vi "WPI_Power Get PDP EnergyPower.vi"(0 "Power Distribution Panel (0)":u8, 7 "Reset Energy?":bool, 11 "error in":errorcluster) -> (6 "Energy (J)":dbl, 8 "Power (W)":dbl, 15 "error out":errorcluster)   [LabVIEW 2017]
doc: "Return the Energy delivered to the robot as well as the recent power delivery."
uses:
  <vilib>/Rock Robotics/WPI/CAN/PDP/WPI_CAN_PDPGlobalOps.ctl
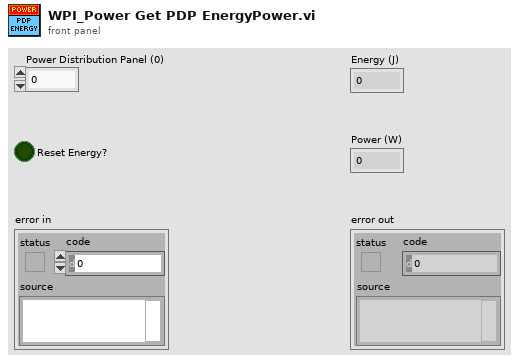
[diagram p1: front panel]
types:
  T1 = typedef "WPI_CAN_PDPGlobalOps.ctl" = enum16{"Write After Receive 0-5", "Write After Receive 6-11", "Write After Receive 12-15", "Write After Receive Energy", "Get All", "Get Commands", "Write Clear Sticky Faults Command", "Write Reset Energy Command", "Write Tare Currents Command", "Write Error", "Write After Receive Faults"}
  T2 = typedef "WPI_CAN_PDPGetAll.ctl" = cluster{"Channel Currents":dbl[], "Battery Voltage":dbl, "Temperature (degrees C)":dbl, "Internal Battery R (Ohms)":dbl, "Energy (J)":dbl, "Power (W)":dbl, "Total Current (A)":dbl, "CAN Error":errorcluster, "Current Faults":bool[], "Battery Voltage Fault":bool, "Temperature Fault":bool, "Hardware Fault":bool}
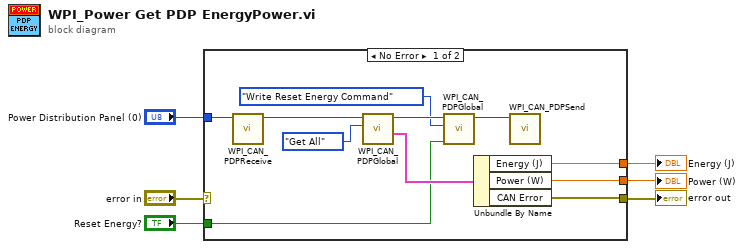
[diagram p0: block diagram]
diagram:
  n1 = case shown="No Error" "error in" {
    selector: "error in" -> [_ w18]
    tunnel: [w8 w18] -> w5
    tunnel: "Power Distribution Panel (0)" -> [w16 _]
    tunnel: [w7 _] -> w2
    tunnel: [w14 _] -> w3
    tunnel: "Reset Energy?" -> [w10 _]
    frame No Error {
      n2 = call <vilib>:"WPI_CAN_PDPReceive.vi"("Power Distribution Panel (0)"=w16) -> ("Power Distribution Panel Out"=w13:u8)  [unwired: 10 in]
      n3 = call <vilib>:"WPI_CAN_PDPGlobal.vi"("Operation"=WPI_CAN_PDPGlobalOps."Get All", "Power Distribution Panel (0)"=w13) -> ("Get All"=w17:T2, "Power Distribution Panel Out"=w12:u8)  [unwired: 7 in, 1 out]
      n4 = call <vilib>:"WPI_CAN_PDPGlobal.vi"("Command"=w10, "Operation"=WPI_CAN_PDPGlobalOps."Write Reset Energy Command", "Power Distribution Panel (0)"=w12) -> ("Power Distribution Panel Out"=w9:u8)  [unwired: 6 in, 2 out]
      n5 = Unbundle By Name(w17) -> ("Energy (J)"=w7:dbl, "Power (W)"=w14:dbl, "CAN Error"=w8:errorcluster)
      n6 = call <vilib>:"WPI_CAN_PDPSend.vi"("Power Distribution Panel (0)"=w9) -> ()  [unwired: 10 in, 1 out]
    }
    frame Error {
    }
  }
  "error out" <- w5
  "Power (W)" <- w3
  "Energy (J)" <- w2
